vi "BATT-ABSOLUTE-Six.vi"(0 "B2":dbl, 1 "A6":dbl, 2 "A3":dbl, 3 "B6":dbl, 4 "B3":dbl, 6 "Comp":dbl, 7 "A4":dbl, 8 "B1":dbl, 9 "B4":dbl, 10 "A2":dbl, 11 "A5":dbl, 12 "A1":dbl, 13 "B5":dbl) -> (14 "Boolean":bool)   [LabVIEW 2016]
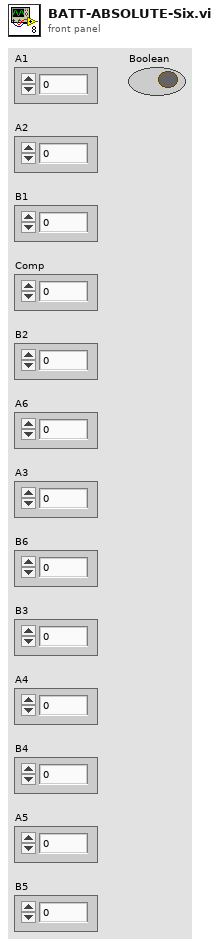
[diagram p1: front panel]
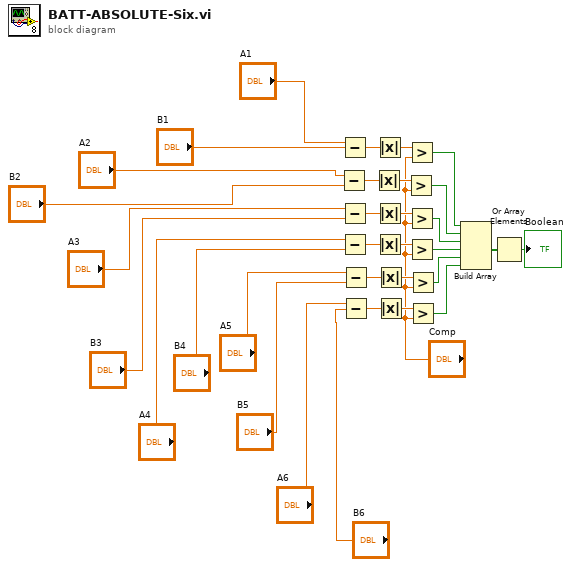
[diagram p0: block diagram]
diagram:
  n1 = Subtract(x="A2", y="B2") -> (x-y=w3:dbl)
  n2 = Subtract(x="A1", y="B1") -> (x-y=w19:dbl)
  n3 = Subtract(x="A3", y="B3") -> (x-y=w5:dbl)
  n4 = Subtract(x="A4", y="B4") -> (x-y=w7:dbl)
  n5 = Subtract(x="A5", y="B5") -> (x-y=w9:dbl)
  n6 = Subtract(x="A6", y="B6") -> (x-y=w11:dbl)
  n7 = Absolute Value(x=w3) -> (abs(x)=w2:dbl)
  n8 = Absolute Value(x=w19) -> (abs(x)=w18:dbl)
  n9 = Absolute Value(x=w5) -> (abs(x)=w4:dbl)
  n10 = Absolute Value(x=w7) -> (abs(x)=w6:dbl)
  n11 = Absolute Value(x=w9) -> (abs(x)=w8:dbl)
  n12 = Absolute Value(x=w11) -> (abs(x)=w10:dbl)
  n13 = Greater?(x=w2, y="Comp") -> (0:w12:bool)
  n14 = Greater?(x=w18, y="Comp") -> (0:w20:bool)
  n15 = Greater?(x=w4, y="Comp") -> (0:w13:bool)
  n16 = Greater?(x=w6, y="Comp") -> (0:w14:bool)
  n17 = Greater?(x=w8, y="Comp") -> (0:w15:bool)
  n18 = Greater?(x=w10, y="Comp") -> (0:w16:bool)
  n19 = Build Array(w20, w12, w13, w14, w15, w16) -> (w17:bool[])
  n20 = Or Array Elements(Boolean array=w17) -> (logical OR=→"Boolean":bool)
